vi "Set Output State.vi"(8 "error in (no error)":cluster{"状态":bool, "代码":i32, "源":string} caption="错误输入（无错误）", 10 "输出状态":bool, 11 "水位控制器输入":refnum<class "Level Controller.lvclass">) -> (0 "error out":cluster{"状态":bool, "代码":i32, "源":string} caption="错误输出", 3 "水位控制器输出":refnum<class "Level Controller.lvclass">)   [LabVIEW 2013, in "Level Controller.lvlib" / "Level Controller.lvclass"]
doc: "该VI负责在水位控制器所监控的变量值高于或低于死区范围时，设定水位控制器的行为。仅当操作模式发生切换时，水位控制器类会调用该VI。当前值高于死区范围时，输入变量“输出状态”为“真”；当前值低于死区范围时，输入变量“输出状态”为“假”。"
uses:
  Level Controller.lvclass
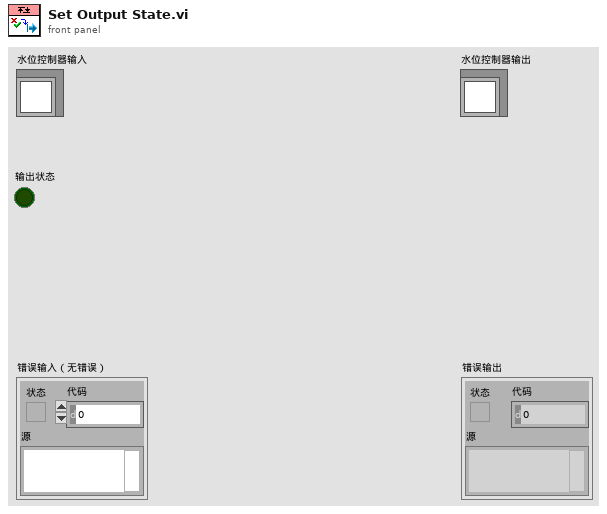
[diagram p1: front panel]
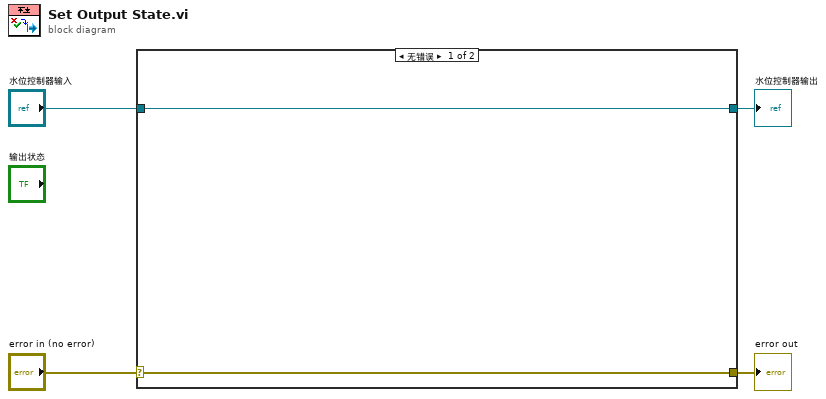
[diagram p0: block diagram]
diagram:
  n1 = case shown="无错误" "error in (no error)" {
    selector: "error in (no error)" -> [w5 w8]
    tunnel: [w5 w8] -> w3
    tunnel: [w6 w7] -> w1
    tunnel: "水位控制器输入" -> [w6 w7]
    frame No Error {
    }
    frame Error {
    }
  }
  "error out" <- w3
  "水位控制器输出" <- w1
